vi "GEOM_GetStrAmps.vi"(10 "args":string) -> (2 "amps":string)   [LabVIEW 2016]
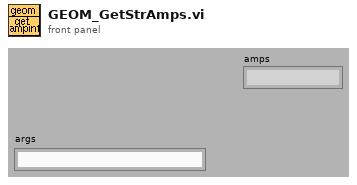
[diagram p1: front panel]
types:
  T1 = typedef "GEOM_Amplifier.ctl" = cluster{"number":i32, "type":T2, "rotated":i16, "fliped":u16, "FPAcoord":cluster{"xstart":i32, "ystart":i32}, "Physical_size":cluster{"columns":i32, "rows":i32}, "predata":cluster{"columns":i32, "rows":i32}, "postdata":cluster{"columns":i32, "rows":i32}, "Req ROIs":T3, "Corr ROI":T3, "Detnumber":i32, "ampID":string, "discard":i32}
  T2 = typedef "GEOM_AmpType.ctl" = u16
  T3 = typedef "GEOM_ROI.ctl" = T4[]
  T4 = typedef "GEOM_Coords.ctl" = cluster{"xstart":u32, "ystart":u32, "xsize":u32, "ysize":u32}
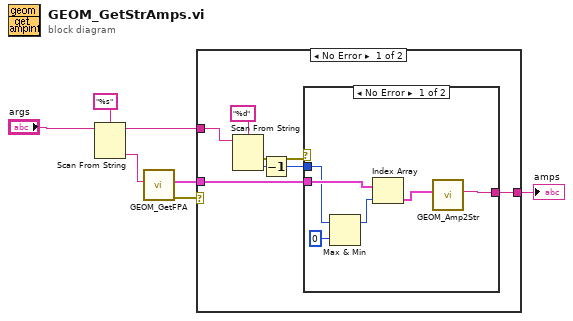
[diagram p0: block diagram]
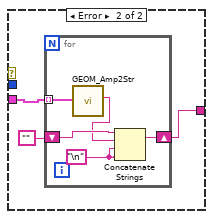
[diagram p2: hidden frame]
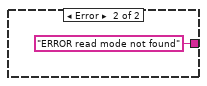
[diagram p3: hidden frame]
diagram:
  n1 = Scan From String(format string="%s", input string="args") -> (remaining string=w2:string, output 1=w5:string)  [unwired: 2 in, 3 out]
  n2 = call "GEOM_GetFPA.vi"("readmode"=w5) -> ("error out"=w4:errorcluster, "amplifiers"=w3:T1[])  [unwired: 2 in, 7 out]
  n3 = case shown="No Error" w4 {
    tunnel: w3 -> [w10 _]
    tunnel: w2 -> [w13 _]
    tunnel: [w9 "ERROR read mode not found" ("resulting string")] -> w1
    frame No Error {
      n4 = Scan From String(format string="%d", input string=w13) -> (error out=w12:errorcluster, output 1=w11:i32)  [unwired: 2 in, 3 out]
      n5 = Decrement(x=w11) -> (x-1=w8:i32)
      n6 = case shown="No Error" w12 {
        tunnel: w8 -> [w17 _]
        tunnel: w10 -> [w20 w23]
        tunnel: [w18 w22] -> w9
        frame No Error {
          n7 = Max & Min(x=w17, y=0) -> (max(x,y)=w15:i32)  [unwired: 1 out]
          n8 = Index Array(array=w20, index=w15) -> (element=w19:T1)
          n9 = call "GEOM_Amp2Str.vi"("amp"=w19) -> ("resulting string"=w18:string)  [unwired: 10 out]
        }
        frame Error {
          n10 = for {
            tunnel: w23 -> [w28] mode=indexing
            shift-right: [w27] -> w22
            shift-left: "" -> [w26]
            w24 = "\n"
            n11 = call "GEOM_Amp2Str.vi"("amp"=w28) -> ("resulting string"=w25:string)  [unwired: 10 out]
            n12 = Concatenate Strings(w26, w25, w24, w24) -> (w27:string)
          }
        }
      }
    }
    frame Error {
    }
  }
  "amps" <- w1
